vi "DAQmx Create AO Channel (sub).vi"(0 "task in":refnum<k21>, 1 "virtual channel name":string, 5 "physical channel name":tag, 7 "output type":i32(ring)=10322 items=["Voltage"=10322, "Current"=10134, "Function Generation"=14750], 11 "error in":errorcluster, 13 "custom scale":tag) -> (4 "task out":refnum<k21>, 10 "channel names":string, 15 "error out":errorcluster)   [LabVIEW 2013]
uses:
  nilvaiu.dll
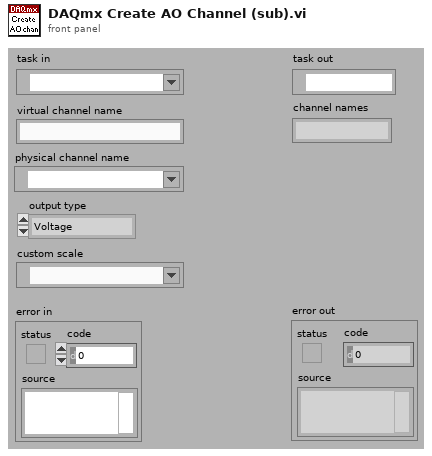
[diagram p1: front panel]
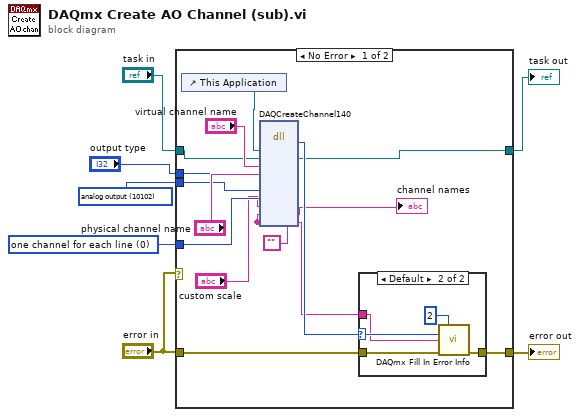
[diagram p0: block diagram]
diagram:
  w2 = 0 items=["one channel for each line", "one channel for all lines"] ("line grouping")
  w4 = 10102 items=["analog input"=10100, "analog output"=10102, "digital input"=10151, "digital output"=10153, "counter input"=10131, "counter output"=10132] ("channel type")
  n1 = case shown="No Error" "error in" {
    tunnel: [w18 w30] -> w7
    tunnel: "error in" -> [w20 w30]
    tunnel: "task in" -> [w9 w29]
    tunnel: "output type" -> [w17 _]
    tunnel: w4 -> [w16 _]
    tunnel: w2 -> [w15 _]
    tunnel: [w10 w29] -> w1
    frame No Error {
      w11 = ""
      n2 = control-ref of="This Application"() -> (w8:refnum<vi>)
      n3 = dll-call lib="nilvaiu.*" fn="DAQCreateChannel140"("lvAppReference"=w8, "taskID"=w9, "virtual channel name"="virtual channel name", "physical channel name"="physical channel name", "measurement type"=w17, "channel type"=w16, "line grouping"=w15, "customScale"="custom scale", "channel names"=w11, "extendedErrorIndo"=w11) -> ("return type"=w19:i32, "taskID"=w10:refnum<k21>, "channel names"=→"channel names":string, "extendedErrorIndo"=w12:string)  [unwired: 10 in, 2 out]
      n4 = case shown="Default" w19 {
        selector: w19 -> [_ w26]
        tunnel: w20 -> [w23 w28]
        tunnel: [w23 w27] -> w18
        tunnel: w12 -> [_ w25]
        frame 0 {
        }
        frame Default {
          n5 = call "DAQmx Fill In Error Info.vi"("depth"=2, "status code"=w26, "extended error info"=w25, "error in"=w28) -> ("error out"=w27:errorcluster)  [unwired: 1 in, 10 out]
        }
      }
    }
    frame Error {
    }
  }
  "error out" <- w7
  "task out" <- w1
